vi "SLIT_generate_script.vi"(1 "Script Type":enum16{"Home", "Change"}(ring), 2 "Current Slit#":i32, 3 "Slit#":i32) -> (0 "script out":T1)   [LabVIEW 2015]
uses:
  SystemUtil/Script.ctl
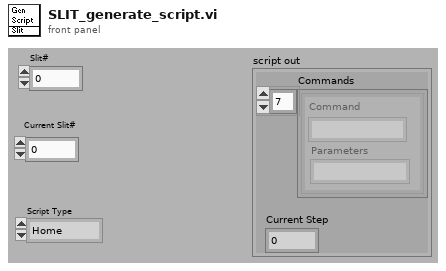
[diagram p1: front panel]
types:
  T1 = typedef "Script.ctl" = cluster{"Current Step":i32, "Commands":cluster{"Command":string, "Parameters":string}[]}
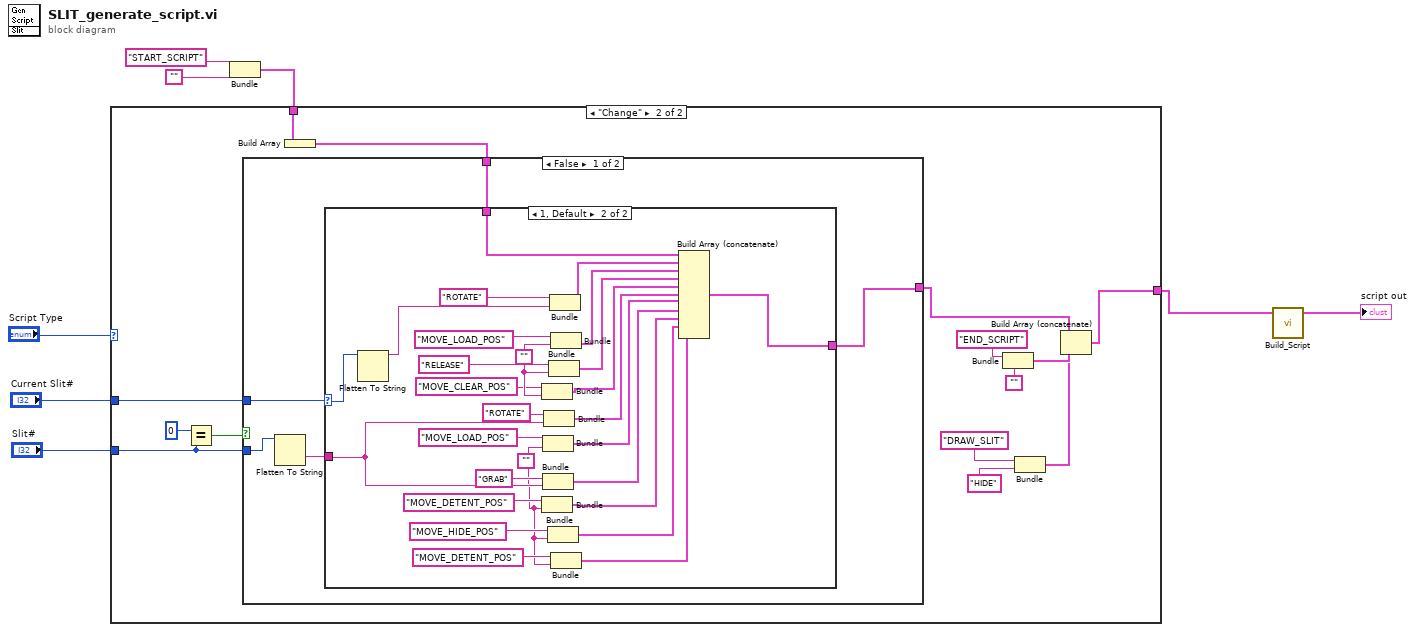
[diagram p0: block diagram]
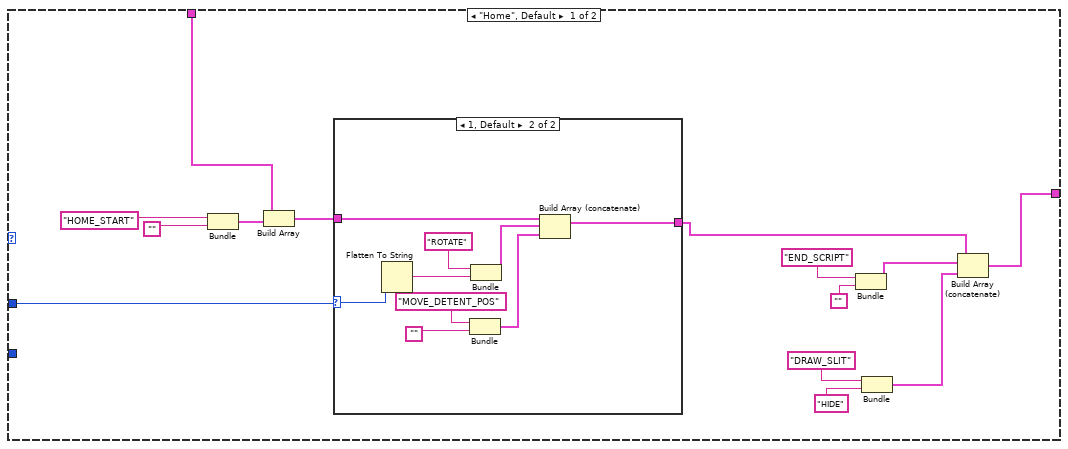
[diagram p2: hidden frame]
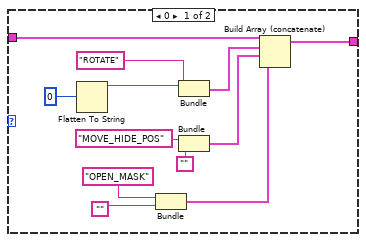
[diagram p3: hidden frame]
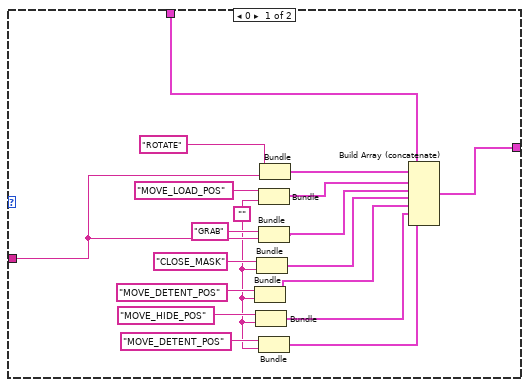
[diagram p4: hidden frame]
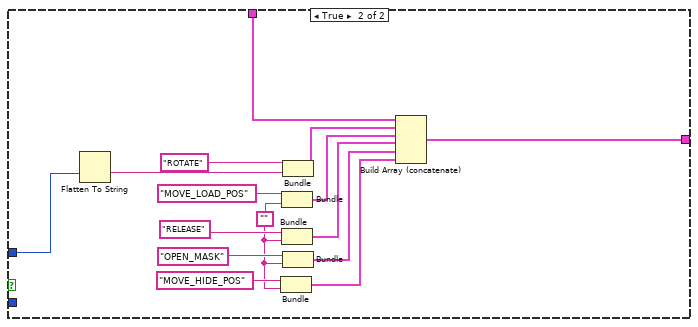
[diagram p5: hidden frame]
diagram:
  n1 = Bundle("START_SCRIPT", "") -> (w2:cluster{string, string})  [unwired: 1 in]
  n2 = case shown="\"Change\"" "Script Type" {
    tunnel: "Current Slit#" -> [w18 w53]
    tunnel: "Slit#" -> [_ w56]
    tunnel: [w12 w47] -> w1
    tunnel: w2 -> [w17 w52]
    frame "Home", Default {
      n3 = Bundle("HOME_START", "") -> (w20:cluster{string, string})  [unwired: 1 in]
      n4 = Build Array(w17, w20) -> (w19:cluster{string, string}[])
      n5 = case shown="1, Default" w18 {
        selector: w18 -> [_ w35]
        tunnel: w19 -> [w30 w41]
        tunnel: [w27 w40] -> w13
        frame 0 {
          n6 = Flatten To String(anything=0) -> (data string=w33:string)  [unwired: 3 in, 2 out]
          n7 = Bundle("OPEN_MASK", "") -> (w23:cluster{string, string})  [unwired: 1 in]
          n8 = Bundle("ROTATE", "data string"=w33) -> (w29:cluster{string, "data string":string})  [unwired: 1 in]
          n9 = Bundle("MOVE_HIDE_POS", "") -> (w28:cluster{string, string})  [unwired: 1 in]
          n10 = Build Array (concatenate)(w30, w29, w28, w23) -> (w27:cluster{string, "data string":string}[])
        }
        frame 1, Default {
          n11 = Flatten To String(anything=w35) -> (data string=w37:string)  [unwired: 3 in, 2 out]
          n12 = Bundle("MOVE_DETENT_POS", "") -> (w39:cluster{string, string})  [unwired: 1 in]
          n13 = Bundle("ROTATE", "data string"=w37) -> (w36:cluster{string, "data string":string})  [unwired: 1 in]
          n14 = Build Array (concatenate)(w41, w36, w39) -> (w40:cluster{string, "data string":string}[])
        }
      }
      n15 = Bundle("END_SCRIPT", "") -> (w16:cluster{string, string})  [unwired: 1 in]
      n16 = Bundle("Command"="DRAW_SLIT", "Parameters"="HIDE") -> (w10:cluster{"Command":string, "Parameters":string})  [unwired: 1 in]
      n17 = Build Array (concatenate)(w13, w16, w10) -> (w12:cluster{"Command":string, "Parameters":string}[])
    }
    frame "Change" {
      n18 = Equal?(x=0 ("y"), y=w56) -> (x = y?=w54:bool)
      n19 = Build Array(w52) -> (w57:cluster{string, string}[])
      n20 = case shown="False" w54 {
        tunnel: w57 -> [w59 w120]
        tunnel: [w60 w119] -> w48
        tunnel: w56 -> [w62 _]
        tunnel: w53 -> [w58 w114]
        frame False {
          n21 = Flatten To String(anything=w62) -> (data string=w61:string)  [unwired: 3 in, 2 out]
          n22 = case shown="1, Default" w58 {
            selector: w58 -> [_ w95]
            tunnel: w61 -> [w68 w97]
            tunnel: [w70 w98] -> w60
            tunnel: w59 -> [w69 w99]
            frame 0 {
              w65 = ""
              n23 = Bundle("MOVE_DETENT_POS", w65) -> (w71:cluster{string, string})  [unwired: 1 in]
              n24 = Bundle("MOVE_HIDE_POS", w65) -> (w64:cluster{string, string})  [unwired: 1 in]
              n25 = Bundle("CLOSE_MASK", w65) -> (w72:cluster{string, string})  [unwired: 1 in]
              n26 = Bundle("MOVE_LOAD_POS", w65) -> (w74:cluster{string, string})  [unwired: 1 in]
              n27 = Bundle("GRAB", "data string"=w68) -> (w73:cluster{string, "data string":string})  [unwired: 1 in]
              n28 = Bundle("MOVE_DETENT_POS", w65) -> (w63:cluster{string, string})  [unwired: 1 in]
              n29 = Bundle("ROTATE", "data string"=w68) -> (w75:cluster{string, "data string":string})  [unwired: 1 in]
              n30 = Build Array (concatenate)(w69, w75, w74, w73, w72, w71, w64, w63) -> (w70:cluster{string, "data string":string}[])
            }
            frame 1, Default {
              w103 = ""
              w83 = ""
              n31 = Flatten To String(anything=w95) -> (data string=w94:string)  [unwired: 3 in, 2 out]
              n32 = Bundle("MOVE_CLEAR_POS", w103) -> (w90:cluster{string, string})  [unwired: 1 in]
              n33 = Bundle("MOVE_DETENT_POS", w83) -> (w86:cluster{string, string})  [unwired: 1 in]
              n34 = Bundle("MOVE_LOAD_POS", w83) -> (w88:cluster{string, string})  [unwired: 1 in]
              n35 = Bundle("GRAB", "data string"=w97) -> (w87:cluster{string, "data string":string})  [unwired: 1 in]
              n36 = Bundle("ROTATE", "data string"=w97) -> (w89:cluster{string, "data string":string})  [unwired: 1 in]
              n37 = Bundle("MOVE_HIDE_POS", w83) -> (w82:cluster{string, string})  [unwired: 1 in]
              n38 = Bundle("RELEASE", w103) -> (w91:cluster{string, string})  [unwired: 1 in]
              n39 = Bundle("ROTATE", "data string"=w94) -> (w93:cluster{string, "data string":string})  [unwired: 1 in]
              n40 = Bundle("MOVE_LOAD_POS", w103) -> (w92:cluster{string, string})  [unwired: 1 in]
              n41 = Bundle("MOVE_DETENT_POS", w83) -> (w81:cluster{string, string})  [unwired: 1 in]
              n42 = Build Array (concatenate)(w99, w93, w92, w91, w90, w89, w88, w87, w86, w82, w81) -> (w98:cluster{string, "data string":string}[])
            }
          }
        }
        frame True {
          w116 = ""
          n43 = Flatten To String(anything=w114) -> (data string=w113:string)  [unwired: 3 in, 2 out]
          n44 = Bundle("MOVE_HIDE_POS", w116) -> (w108:cluster{string, string})  [unwired: 1 in]
          n45 = Bundle("MOVE_LOAD_POS", w116) -> (w111:cluster{string, string})  [unwired: 1 in]
          n46 = Bundle("RELEASE", w116) -> (w110:cluster{string, string})  [unwired: 1 in]
          n47 = Bundle("ROTATE", "data string"=w113) -> (w112:cluster{string, "data string":string})  [unwired: 1 in]
          n48 = Bundle("OPEN_MASK", w116) -> (w109:cluster{string, string})  [unwired: 1 in]
          n49 = Build Array (concatenate)(w120, w112, w111, w110, w109, w108) -> (w119:cluster{string, "data string":string}[])
        }
      }
      n50 = Bundle("END_SCRIPT", "") -> (w51:cluster{string, string})  [unwired: 1 in]
      n51 = Bundle("Command"="DRAW_SLIT", "Parameters"="HIDE") -> (w44:cluster{"Command":string, "Parameters":string})  [unwired: 1 in]
      n52 = Build Array (concatenate)(w48, w51, w44) -> (w47:cluster{"Command":string, "Parameters":string}[])
    }
  }
  n53 = call "Build_Script.vi"("Commands"=w1) -> ("script out"=→"script out":T1)  [unwired: 4 in]
